vi "read voltage map.vi"(8 "error in (no error)":errorcluster, 11 "BMC in":refnum<class "BMC.lvclass">) -> (0 "error out":errorcluster, 2 "1x160 Voltage Map":dbl[](array[numeric]), 3 "BMC out":refnum<class "BMC.lvclass">)   [LabVIEW 2012, in "BMC.lvclass"]
uses:
  BMC.lvclass
  BMC.lvclass/BMC.ctl
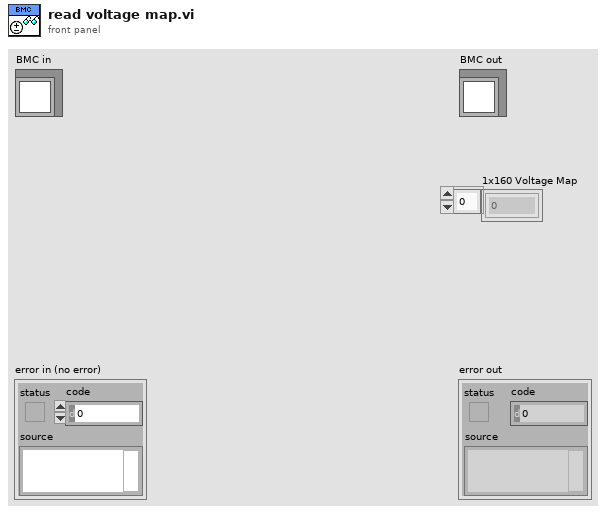
[diagram p1: front panel]
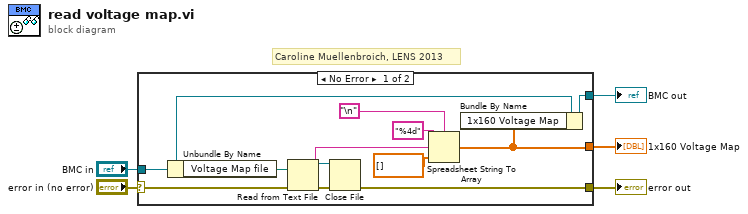
[diagram p0: block diagram]
diagram:
  # "Caroline Muellenbroich, LENS 2013"
  n1 = case shown="No Error" "error in (no error)" {
    selector: "error in (no error)" -> [w12 w19]
    tunnel: [w10 w19] -> w4
    tunnel: [w13 w18] -> w2
    tunnel: "BMC in" -> [w14 w18]
    tunnel: [w8 _] -> w1
    frame No Error {
      n2 = Unbundle By Name(w14) -> ("Voltage Map file"=w7:path)
      n3 = Read from Text File(file (use dialog)=w7, error in=w12) -> (refnum out=w15:refnum<file>, text=w17:string, error out=w11:errorcluster)  [unwired: 3 out]
      n4 = Close File(refnum=w15, error in=w11) -> (error out=w10:errorcluster)  [unwired: 1 out]
      n5 = Spreadsheet String To Array(delimiter (Tab)="\n", format string="%4d", spreadsheet string=w17, array type (2D Dbl)=dbl[] [] ("run time Cluster.1x160  Voltage Map")) -> (array=w8:dbl[])
      n6 = Bundle By Name(cluster=w14, "1x160 Voltage Map"=w8) -> (w13:refnum<class "BMC.lvclass">)
    }
    frame Error {
    }
  }
  "error out" <- w4
  "BMC out" <- w2
  "1x160 Voltage Map" <- w1
